vi "ParameterSweeper.vi"() -> ()   [LabVIEW 2019]
uses:
  <vilib>/regexp/Match Regular Expression.xnode
panel:
  out "status 2":bool
  out "status":bool
  in  "Swap":bool
  out "Period (s)":dbl=16.0
  out "Value 2":dbl
  out "Value":dbl=2.0
  out "steps 2":dbl=4.0
  out "steps":dbl=4.0
  in  "Setting":T1={"interval (s)"=1.0, "Second Dimension"=FALSE, "start"=0.0, "stop"=2.0, "step"=1.0, "round trip"=TRUE, "vi"="", "ctrl"="", "start 2"=0.0, "stop 2"=2.0, "step 2"=1.0, "round trip 2"=FALSE, "vi 2"="", "ctrl 2"=""} {"interval (s)" min=0.1 max=100.0}
  out "Slip Count":i32
  in  "Record Sync":bool
  in  "Sweep Start":bool
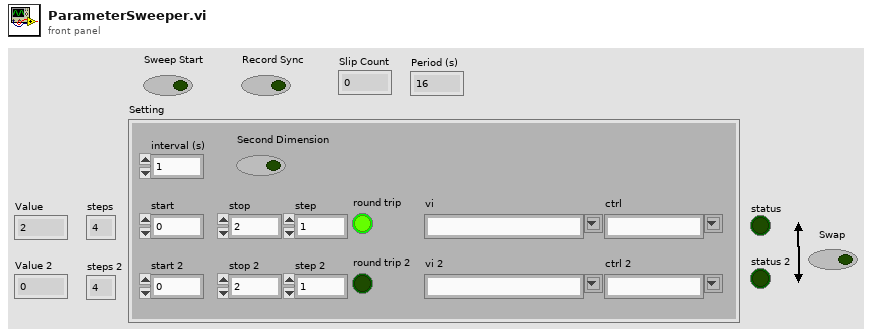
[diagram p1: front panel]
types:
  T1 = cluster{"interval (s)":dbl, "Second Dimension":bool, "start":dbl, "stop":dbl, "step":dbl, "round trip":bool, "vi":string, "ctrl":string, "start 2":dbl, "stop 2":dbl, "step 2":dbl, "round trip 2":bool, "vi 2":string, "ctrl 2":string}
  T2 = enum32{"Invalid", "Standard", "Closed", "Hidden", "Minimized", "Maximized"}
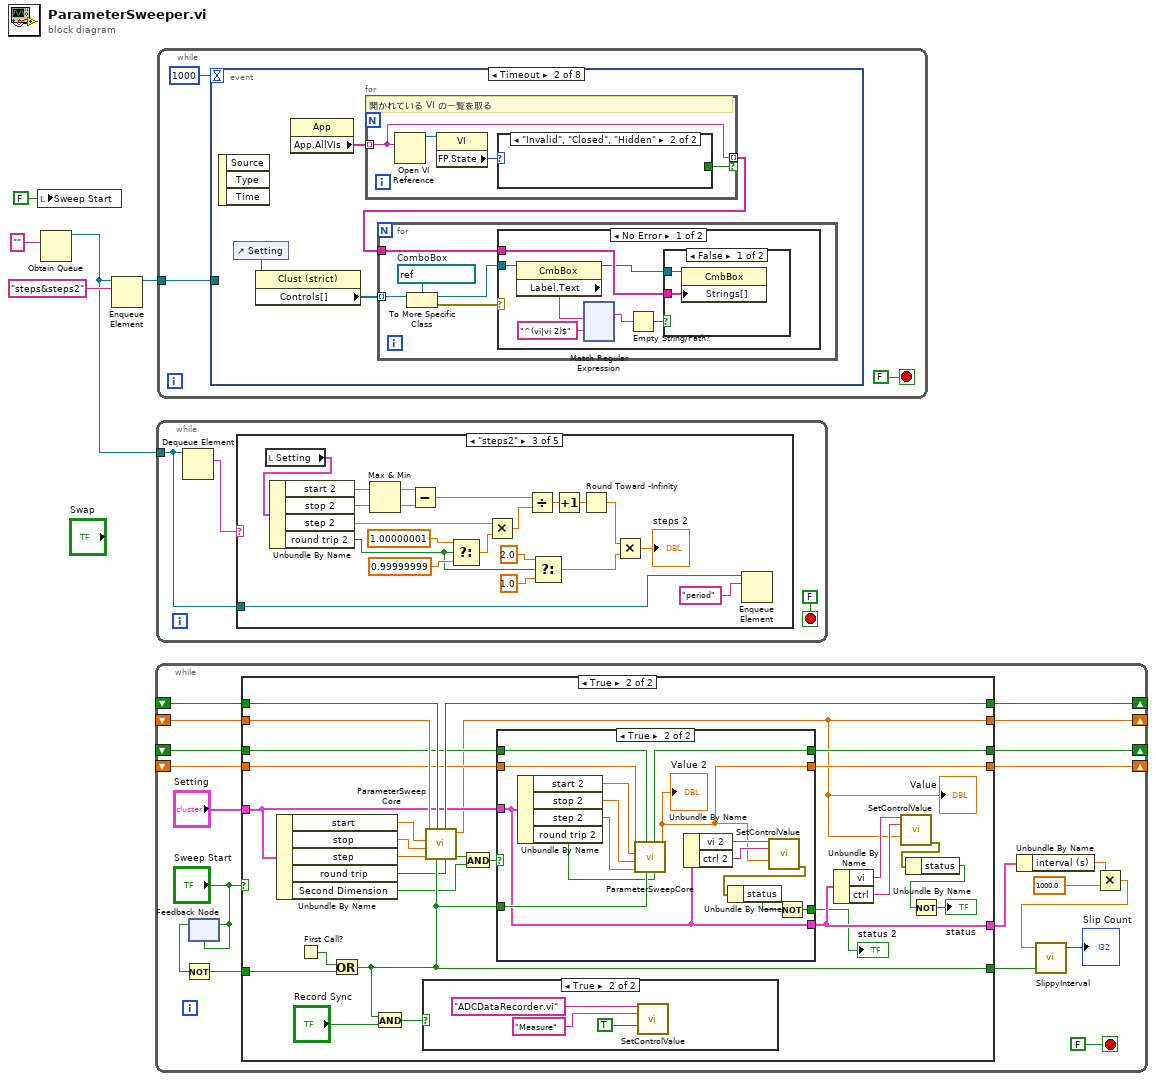
[diagram p0: block diagram]
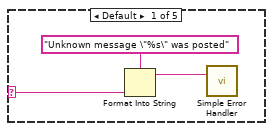
[diagram p2: hidden frame]
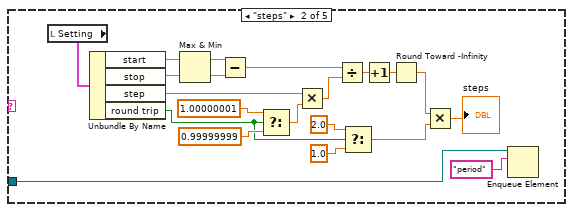
[diagram p3: hidden frame]
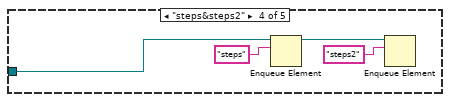
[diagram p4: hidden frame]
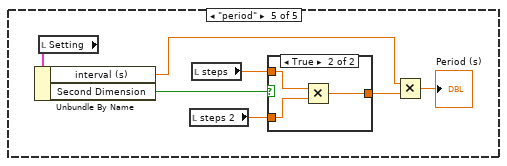
[diagram p5: hidden frame]
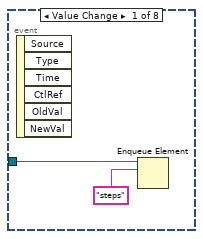
[diagram p7: hidden frame]
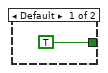
[diagram p8: hidden frame]
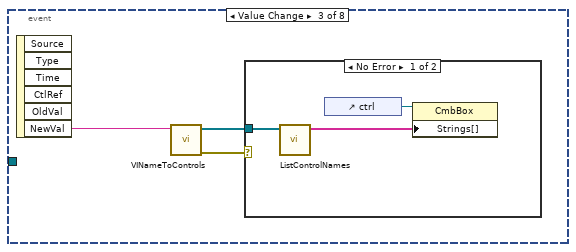
[diagram p11: hidden frame]
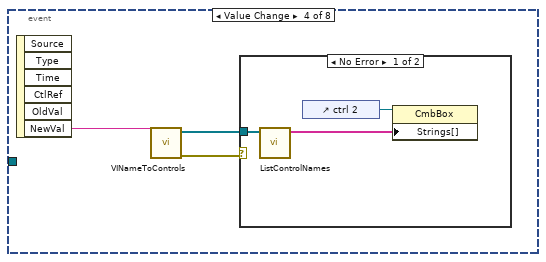
[diagram p13: hidden frame]
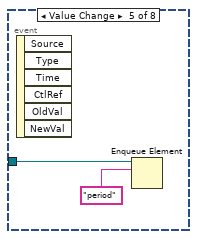
[diagram p15: hidden frame]
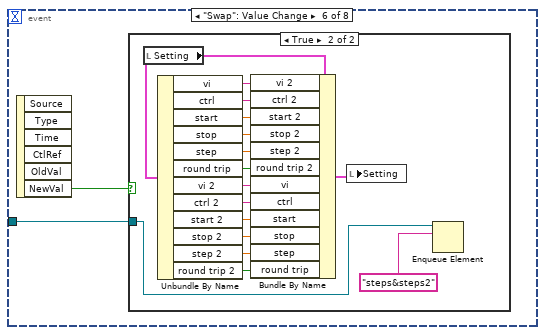
[diagram p16: hidden frame]
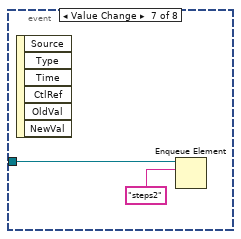
[diagram p18: hidden frame]
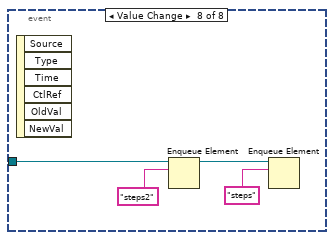
[diagram p19: hidden frame]
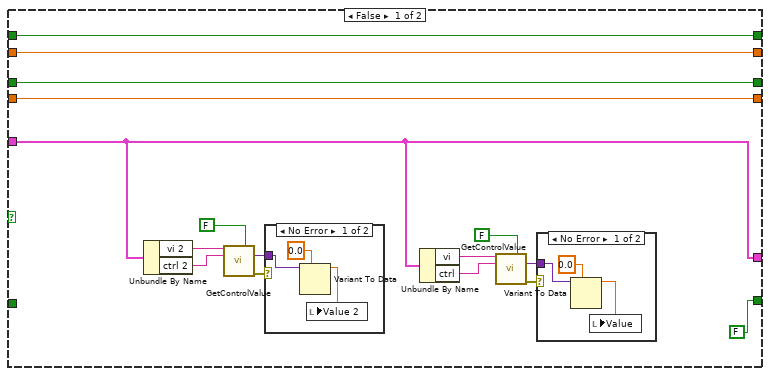
[diagram p20: hidden frame]
diagram:
  n1 = local write "Sweep Start"(FALSE ("Sweep Start")) -> ()
  n2 = Obtain Queue(element data type="") -> (queue out=w1:refnum<queue>)  [unwired: 4 in, 2 out]
  n3 = Enqueue Element(queue=w1, element="steps&steps2") -> (queue out=w3:refnum<queue>)  [unwired: 2 in, 2 out]
  n4 = while {
    shift-right: [w7] -> _
    shift-left: _ -> [w24]
    shift-right: [w22] -> _
    shift-left: _ -> [w23]
    shift-right: [w21] -> _
    shift-left: _ -> [w20]
    shift-right: [w6] -> _
    shift-left: _ -> [w19]
    stop <- FALSE stop-if-true
    n5 = feedback #1("Sweep Start") -> (w12:bool)
    n6 = Not(x=w12) -> (.not. x?=w11:bool)
    n7 = feedback-in #1("Sweep Start") -> ()
    n8 = case shown="True" "Sweep Start" {
      tunnel: w24 -> [w38 w74]
      tunnel: w23 -> [w39 w73]
      tunnel: [w39 w72] -> w22
      tunnel: [w37 w71] -> w21
      tunnel: [w36 w70] -> w6
      tunnel: w20 -> [w37 w69]
      tunnel: w19 -> [w36 w68]
      tunnel: [w38 w47] -> w7
      tunnel: [FALSE w64] -> w17
      tunnel: w11 -> [_ w48]
      tunnel: "Setting" -> [w28 w56]
      tunnel: [w28 w55] -> w9
      frame False {
        n9 = Unbundle By Name(w28) -> ("vi 2"=w35:string, "ctrl 2"=w34:string)
        n10 = call "GetControlValue.vi"("vi"=w35, "UseEnum (true)"=FALSE, "ctrl"=w34) -> ("value"=w26:variant, "error out"=w33:errorcluster)  [unwired: 10 in, 1 out]
        n11 = case shown="No Error" w33 {
          tunnel: w26 -> [w46 _]
          frame No Error {
            n12 = Variant To Data(type=0.0 ("Value 2"), Variant=w46) -> (data=w44:dbl)  [unwired: 1 in, 1 out]
            n13 = local write "Value 2"(w44) -> ()
          }
          frame Error {
          }
        }
        n14 = Unbundle By Name(w28) -> ("vi"=w31:string, "ctrl"=w30:string)
        n15 = call "GetControlValue.vi"("vi"=w31, "UseEnum (true)"=FALSE, "ctrl"=w30) -> ("value"=w25:variant, "error out"=w29:errorcluster)  [unwired: 10 in, 1 out]
        n16 = case shown="No Error" w29 {
          tunnel: w25 -> [w41 _]
          frame No Error {
            n17 = Variant To Data(type=0.0 ("Value 2"), Variant=w41) -> (data=w42:dbl)  [unwired: 1 in, 1 out]
            n18 = local write "Value"(w42) -> ()
          }
          frame Error {
          }
        }
      }
      frame True {
        n19 = Unbundle By Name(w56) -> ("start"=w62:dbl, "stop"=w61:dbl, "step"=w60:dbl, "round trip"=w59:bool, "Second Dimension"=w58:bool)
        n20 = First Call?() -> (First Call?: T/F=w49:bool)
        n21 = Or(x=w49, y=w48) -> (x .or. y?=w64:bool)
        n22 = And(x=w64, y="Record Sync") -> (x .and. y?=w63:bool)
        n23 = case shown="True" w63 {
          frame False {
          }
          frame True {
            n24 = call "SetControlValue.vi"("vi"="ADCDataRecorder.vi", "ctrl"="Measure", "Value"=TRUE) -> ()  [unwired: 12 in, 1 out]
          }
        }
        n25 = call "ParameterSweepCore.vi"("Round Trip"=w59, "Initialize"=w64, "Backward in"=w73, "Step"=w60, "To"=w61, "From"=w62, "Value in"=w74) -> ("New Sweep"=w66:bool, "Value out"=w47:dbl, "Backward out"=w72:bool)  [unwired: 2 in]
        "Value" <- w47
        n26 = And(x=w66, y=w58) -> (x .and. y?=w67:bool)
        n27 = case shown="True" w67 {
          tunnel: [w80 w95] -> w71
          tunnel: [w79 w81] -> w70
          tunnel: w69 -> [w80 w94]
          tunnel: w68 -> [w79 w93]
          tunnel: w64 -> [_ w92]
          tunnel: w56 -> [w78 w85]
          tunnel: [w78 w85] -> w55
          tunnel: [_ w82] -> w51
          frame False {
          }
          frame True {
            n28 = Unbundle By Name(w85) -> ("start 2"=w91:dbl, "stop 2"=w90:dbl, "step 2"=w89:dbl, "round trip 2"=w88:bool)
            n29 = call "ParameterSweepCore.vi"("Round Trip"=w88, "Initialize"=w92, "Backward in"=w94, "Step"=w89, "To"=w90, "From"=w91, "Value in"=w93) -> ("Value out"=w81:dbl, "Backward out"=w95:bool)  [unwired: 2 in, 1 out]
            "Value 2" <- w81
            n30 = Unbundle By Name(w85) -> ("vi 2"=w87:string, "ctrl 2"=w86:string)
            n31 = call "SetControlValue.vi"("vi"=w87, "ctrl"=w86, "Value"=w81) -> ("error out"=w84:errorcluster)  [unwired: 12 in]
            n32 = Unbundle By Name(w84) -> ("status"=w83:bool)
            n33 = Not(x=w83) -> (.not. x?=w82:bool)
          }
        }
        "status 2" <- w51
        n34 = Unbundle By Name(w55) -> ("vi"=w57:string, "ctrl"=w50:string)
        n35 = call "SetControlValue.vi"("vi"=w57, "ctrl"=w50, "Value"=w47) -> ("error out"=w54:errorcluster)  [unwired: 12 in]
        n36 = Unbundle By Name(w54) -> ("status"=w53:bool)
        n37 = Not(x=w53) -> (.not. x?=→"status":bool)
      }
    }
    n38 = Unbundle By Name(w9) -> ("interval (s)"=w8:dbl)
    n39 = Multiply(x=w8, y=1000.0) -> (x*y=w15:dbl)
    n40 = call "SlippyInterval.vi"("Reset"=w17, "Interval (ms)"=w15) -> ("Slip Count"=→"Slip Count":i32)  [unwired: 1 in, 2 out]
  }
  n41 = while {
    tunnel: w1 -> [w96]
    stop <- FALSE stop-if-true
    n42 = Dequeue Element(queue=w96) -> (element=w98:string)  [unwired: 2 in, 3 out]
    n43 = case shown="\"steps2\"" w98 {
      selector: w98 -> [w100 _ _ _ _]
      tunnel: w96 -> [_ w102 w142 w146 _]
      frame Default {
        n44 = Format Into String(format string="Unknown message \"%s\" was posted", w100) -> (resulting string=w99:string)  [unwired: 2 in, 1 out]
        n45 = call <vilib>:"Simple Error Handler.vi"("error source (\" \")"=w99) -> ()  [unwired: 4 in, 5 out]
      }
      frame "steps" {
        n46 = local read "Setting"() -> (w103:T1)
        n47 = Unbundle By Name(w103) -> ("start"=w113:dbl, "stop"=w112:dbl, "step"=w117:dbl, "round trip"=w104:bool)
        n48 = Max & Min(x=w113, y=w112) -> (max(x,y)=w111:dbl, min(x,y)=w110:dbl)
        n49 = Subtract(x=w111, y=w110) -> (x-y=w119:dbl)
        n50 = Select(t=1.00000001 ("y"), s=w104, f=0.99999999 ("y")) -> (s? t:f=w106:dbl)
        n51 = Multiply(x=w117, y=w106) -> (x*y=w120:dbl)
        n52 = Divide(x=w119, y=w120) -> (x/y=w105:dbl)
        n53 = Select(t=2.0, s=w104, f=1.0) -> (s? t:f=w121:dbl)
        n54 = Increment(x=w105) -> (x+1=w122:dbl)
        n55 = Round Toward -Infinity(1:w122) -> (0:w116:dbl)
        n56 = Multiply(x=w116, y=w121) -> (x*y=→"steps":dbl)
        n57 = Enqueue Element(queue=w102, element="period") -> ()  [unwired: 2 in, 3 out]
      }
      frame "steps2" {
        n58 = local read "Setting"() -> (w141:T1)
        n59 = Unbundle By Name(w141) -> ("start 2"=w124:dbl, "stop 2"=w125:dbl, "step 2"=w126:dbl, "round trip 2"=w127:bool)
        n60 = Max & Min(x=w124, y=w125) -> (max(x,y)=w134:dbl, min(x,y)=w133:dbl)
        n61 = Subtract(x=w134, y=w133) -> (x-y=w137:dbl)
        n62 = Select(t=1.00000001 ("y"), s=w127, f=0.99999999 ("y")) -> (s? t:f=w129:dbl)
        n63 = Multiply(x=w126, y=w129) -> (x*y=w138:dbl)
        n64 = Divide(x=w137, y=w138) -> (x/y=w128:dbl)
        n65 = Select(t=2.0, s=w127, f=1.0) -> (s? t:f=w139:dbl)
        n66 = Increment(x=w128) -> (x+1=w140:dbl)
        n67 = Round Toward -Infinity(1:w140) -> (0:w135:dbl)
        n68 = Multiply(x=w135, y=w139) -> (x*y=→"steps 2":dbl)
        n69 = Enqueue Element(queue=w142, element="period") -> ()  [unwired: 2 in, 3 out]
      }
      frame "steps&steps2" {
        n70 = Enqueue Element(queue=w146, element="steps") -> (queue out=w145:refnum<queue>)  [unwired: 2 in, 2 out]
        n71 = Enqueue Element(queue=w145, element="steps2") -> ()  [unwired: 2 in, 3 out]
      }
      frame "period" {
        n72 = local read "Setting"() -> (w148:T1)
        n73 = Unbundle By Name(w148) -> ("interval (s)"=w151:dbl, "Second Dimension"=w154:bool)
        n74 = local read "steps 2"() -> (w152:dbl)
        n75 = local read "steps"() -> (w153:dbl)
        n76 = case shown="True" w154 {
          tunnel: w153 -> [w155 w158]
          tunnel: w152 -> [_ w157]
          tunnel: [w155 w156] -> w150
          frame False {
          }
          frame True {
            n77 = Multiply(x=w158, y=w157) -> (x*y=w156:dbl)
          }
        }
        n78 = Multiply(x=w151, y=w150) -> (x*y=→"Period (s)":dbl)
      }
    }
  }
  n79 = while {
    tunnel: w3 -> [w160]
    stop <- FALSE stop-if-true
    n80 = event shown="[1] Timeout" {
      selector: _ -> [_ _ _ _ _ _ _ _]
      dyn-events: _ -> [_ _ _ _ _ _ _ _]
      timeout: 1000 -> [_ _ _ _ _ _ _ _]
      tunnel: w160 -> [w163 _ _ _ w317 w318 w336 w338]
      event "Setting.start", "Setting.stop", "Setting.step", "Setting.round trip": Value Change {
        n81 = event-data() -> ()  [unwired: 1 in, 6 out]
        n82 = Enqueue Element(queue=w163, element="steps") -> ()  [unwired: 2 in, 3 out]
      }
      event Timeout {
        n83 = event-data() -> ()  [unwired: 1 in, 3 out]
        n84 = control-ref of="Setting"() -> (w167:refnum<vi>)
        n85 = property class="Clust (strict)"(reference=w167) -> ("Controls[]"=w166:refnum<vi>[])  [unwired: 1 in, 2 out]
        n86 = property class="App"() -> ("App.AllVIs"=w165:string[])  [unwired: 2 in, 2 out]
        n87 = for {
          tunnel: w165 -> [w168] mode=indexing
          tunnel: [w168] -> w164 mode=indexing if=w169
          # "開かれている VI の一覧を取る"
          n88 = Open VI Reference(vi path=w168) -> (vi reference=w171:refnum<vi>)  [unwired: 5 in, 1 out]
          n89 = property class="VI"(reference=w171) -> ("FP.State"=w170:T2)  [unwired: 1 in, 2 out]
          n90 = case shown="\"Invalid\", \"Closed\", \"Hidden\"" w170 {
            tunnel: [TRUE _] -> w169
            frame Default {
            }
            frame "Invalid", "Closed", "Hidden" {
            }
          }
        }
        n91 = for {
          tunnel: w166 -> [w177] mode=indexing
          tunnel: w164 -> [w173]
          w176 = refnum<vi> refnum  # ComboBox
          n92 = To More Specific Class(target class=w176, reference=w177) -> (specific class reference=w174:refnum<vi>, error out=w175:errorcluster)  [unwired: 1 in]
          n93 = case shown="No Error" w175 {
            tunnel: w174 -> [w183 _]
            tunnel: w173 -> [w184 _]
            frame No Error {
              n94 = property class="CmbBox"(reference=w183) -> (reference out=w182:refnum<vi>, "Label.Text"=w181:string)  [unwired: 1 in, 1 out]
              n95 = xnode "Match Regular Expression"("input string"="^(vi|vi 2)$", "regular expression"=w181) -> ("whole match"=w179:string)  [unwired: 4 in, 4 out]
              n96 = Empty String/Path?(string/path=w179) -> (empty?=w178:bool)
              n97 = case shown="False" w178 {
                tunnel: w184 -> [w186 _]
                tunnel: w182 -> [w185 _]
                frame False {
                  n98 = property class="CmbBox"(reference=w185, "Strings[]"=w186) -> ()  [unwired: 1 in, 2 out]
                }
                frame True {
                }
              }
            }
            frame Error {
            }
          }
        }
      }
      event "Setting.vi": Value Change {
        n99 = event-data() -> ("NewVal"=w306:string)  [unwired: 1 in, 5 out]
        n100 = call "VINameToControls.vi"("vi"=w306) -> ("error out"=w304:errorcluster, "FlattenControls[]"=w305:refnum<vi>[])  [unwired: 8 in, 1 out]
        n101 = case shown="No Error" w304 {
          tunnel: w305 -> [w307 _]
          frame No Error {
            n102 = call "ListControlNames.vi"("FlattenControls[]"=w307) -> ("Array"=w308:string[])  [unwired: 9 in, 1 out]
            n103 = control-ref of="ctrl"() -> (w309:refnum<vi>)
            n104 = property class="CmbBox"(reference=w309, "Strings[]"=w308) -> ()  [unwired: 1 in, 2 out]
          }
          frame Error {
          }
        }
      }
      event "Setting.vi 2": Value Change {
        n105 = event-data() -> ("NewVal"=w311:string)  [unwired: 1 in, 5 out]
        n106 = call "VINameToControls.vi"("vi"=w311) -> ("error out"=w310:errorcluster, "FlattenControls[]"=w312:refnum<vi>[])  [unwired: 8 in, 1 out]
        n107 = case shown="No Error" w310 {
          tunnel: w312 -> [w314 _]
          frame No Error {
            n108 = call "ListControlNames.vi"("FlattenControls[]"=w314) -> ("Array"=w315:string[])  [unwired: 9 in, 1 out]
            n109 = control-ref of="ctrl 2"() -> (w313:refnum<vi>)
            n110 = property class="CmbBox"(reference=w313, "Strings[]"=w315) -> ()  [unwired: 1 in, 2 out]
          }
          frame Error {
          }
        }
      }
      event "Setting.Second Dimension": Value Change {
        n111 = event-data() -> ()  [unwired: 1 in, 6 out]
        n112 = Enqueue Element(queue=w317, element="period") -> ()  [unwired: 2 in, 3 out]
      }
      event "Swap": Value Change {
        n113 = event-data() -> ("NewVal"=w319:bool)  [unwired: 1 in, 5 out]
        n114 = case shown="True" w319 {
          tunnel: w318 -> [_ w335]
          frame False {
          }
          frame True {
            n115 = local read "Setting"() -> (w334:T1)
            n116 = Unbundle By Name(w334) -> ("vi"=w333:string, "ctrl"=w332:string, "start"=w331:dbl, "stop"=w330:dbl, "step"=w329:dbl, "round trip"=w328:bool, "vi 2"=w327:string, "ctrl 2"=w326:string, "start 2"=w325:dbl, "stop 2"=w324:dbl, "step 2"=w323:dbl, "round trip 2"=w322:bool)
            n117 = Bundle By Name(cluster=w334, "vi 2"=w333, "ctrl 2"=w332, "start 2"=w331, "stop 2"=w330, "step 2"=w329, "round trip 2"=w328, "vi"=w327, "ctrl"=w326, "start"=w325, "stop"=w324, "step"=w323, "round trip"=w322) -> (w321:T1)
            n118 = local write "Setting"(w321) -> ()
            n119 = Enqueue Element(queue=w335, element="steps&steps2") -> ()  [unwired: 2 in, 3 out]
          }
        }
      }
      event "Setting.start 2", "Setting.stop 2", "Setting.step 2", "Setting.round trip 2": Value Change {
        n120 = event-data() -> ()  [unwired: 1 in, 6 out]
        n121 = Enqueue Element(queue=w336, element="steps2") -> ()  [unwired: 2 in, 3 out]
      }
      event "Setting.interval (s)": Value Change {
        n122 = event-data() -> ()  [unwired: 1 in, 6 out]
        n123 = Enqueue Element(queue=w338, element="steps2") -> (queue out=w339:refnum<queue>)  [unwired: 2 in, 2 out]
        n124 = Enqueue Element(queue=w339, element="steps") -> ()  [unwired: 2 in, 3 out]
      }
    }
  }
